vi "TP 4.1 (programable).vi"() -> ()   [LabVIEW 2013]
uses:
  <vilib>/gmath/statdist.llb/Normal Inverse CDF.vi
  <vilib>/gmath/NI_Gmath.lvlib
panel:
  in  "N promedio":dbl=10.0
  out "Waveform Chart":cluster{"x":dbl, dbl}(graph)
  in  "stop":bool
  in  "Nivel de ruido":dbl=2.0
  in  "Medicion":dbl=10.0
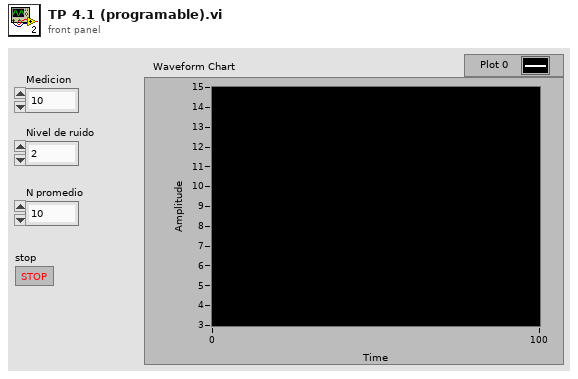
[diagram p1: front panel]
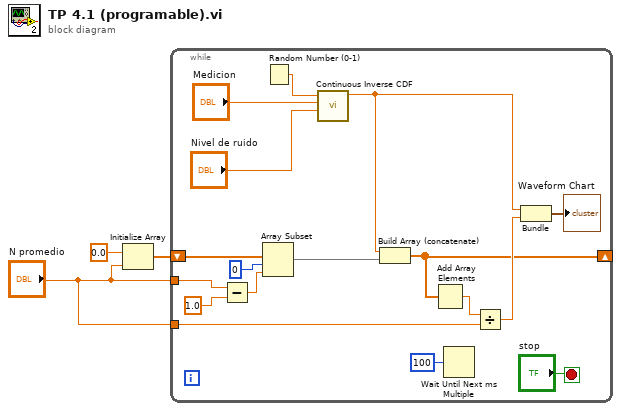
[diagram p0: block diagram]
diagram:
  n1 = Initialize Array(0.0 ("element"), "N promedio") -> (w2:dbl[])
  n2 = while {
    shift-right: [w5] -> _
    shift-left: w2 -> [w13]
    tunnel: "N promedio" -> [w11]
    tunnel: "N promedio" -> [w7]
    stop <- "stop" stop-if-true
    n3 = Subtract(x=w11, y=1.0) -> (x-y=w9:dbl)
    n4 = Array Subset(array=w13, index=0, length=w9) -> (w8:dbl[])
    n5 = Random Number (0-1)() -> (number: 0 to 1=w18:dbl)
    n6 = call-poly <vilib>:"Continuous Inverse CDF.vi"("std"="Nivel de ruido", "mean"="Medicion", "cdf(x)"=w18) -> ("x"=w4:dbl)  [unwired: 7 in, 1 out]
    n7 = Build Array (concatenate)(w4, w8) -> (w5:dbl[])
    n8 = Add Array Elements(numeric array=w5) -> (sum=w6:dbl)
    n9 = Wait Until Next ms Multiple(millisecond multiple=u32 100) -> ()  [unwired: 1 out]
    n10 = Divide(x=w6, y=w7) -> (x/y=w17:dbl)
    n11 = Bundle("x"=w4, w17) -> (→"Waveform Chart":cluster{"x":dbl, dbl})  [unwired: 1 in]
  }
